vi "Read (Single Line).vi"(8 "error in":errorcluster, 11 "VISA resource name":refnum<visa-resource-name>) -> (0 "error out":errorcluster, 2 "Line":string, 3 "VISA resource name 2":refnum<visa-resource-name>)   [LabVIEW 2021, in "Zaber A Series.lvlib"]
doc: "Reads a single line from the VISA resource. Lines are assumed to be delimited by the carriage return and line feed characters"
uses:
  Zaber A Series.lvlib
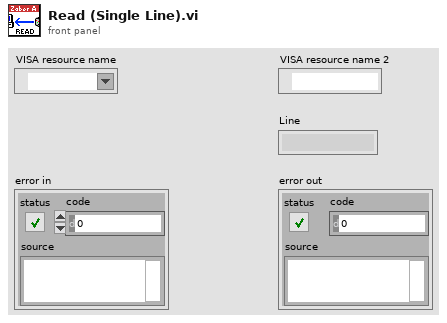
[diagram p1: front panel]
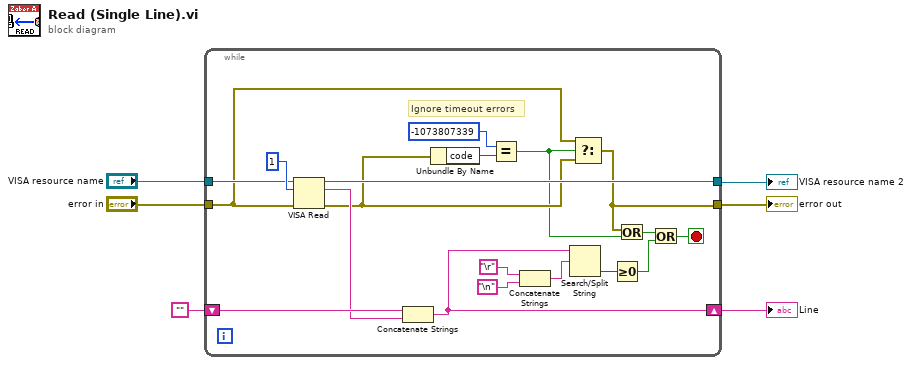
[diagram p0: block diagram]
diagram:
  n1 = while {
    tunnel: "error in" -> [w14]
    tunnel: "VISA resource name" -> [w18]
    tunnel: [w10] -> w6
    tunnel: [w25] -> w5
    shift-right: [w15] -> w3
    shift-left: "" -> [w24]
    stop <- w22 stop-if-true
    # "Ignore timeout errors"
    n2 = VISA Read(VISA resource name=w18, byte count=u32 1, error in (no error)=w14) -> (VISA resource name out=w25:refnum<visa-resource-name>, read buffer=w17:string, error out=w13:errorcluster)  [unwired: 1 out]
    n3 = Concatenate Strings(w24, w17) -> (w15:string)
    n4 = Unbundle By Name(w13) -> ("code"=w8:i32)
    n5 = Equal?(x=-1073807339 ("y"), y=w8) -> (x = y?=w9:bool)
    n6 = Concatenate Strings("\r", "\n") -> (w21:string)
    n7 = Search/Split String(string=w15, search string/char (-)=w21) -> (offset of match=w19:i32)  [unwired: 1 in, 2 out]
    n8 = Select(t=w14, s=w9, f=w13) -> (s? t:f=w10:errorcluster)
    n9 = Greater Or Equal To 0?(x=w19) -> (x >= 0?=w12:bool)
    n10 = Or(x=w10, y=w9) -> (x .or. y?=w11:bool)
    n11 = Or(x=w11, y=w12) -> (x .or. y?=w22:bool)
  }
  "VISA resource name 2" <- w5
  "error out" <- w6
  "Line" <- w3
